vi "Unpack for gRPC.vi"(8 "error in":errorcluster, 9 "configuration / results":enum16{"Configuration", "Results"}(ring), 10 "any":T1, 11 "measurement customizations in":refnum<class "Measurement Plugin.lvclass">) -> (0 "error out":errorcluster, 2 "data value":variant, 3 "measurement customizations out":refnum<class "Measurement Plugin.lvclass">)   [LabVIEW 2021, in "Short-Circuit.lvlib" / "Measurement Plugin.lvclass"]
uses:
  Measurement Plugin.lvclass
  <vilib>/gRPC/LabVIEW gRPC Library/Shared/Any.ctl
  C:/Program Files/National Instruments/LabVIEW 2021/vi.lib/Plug-In SDKs/Measurements/Measurement Plugin Service/Measurement Plugin Service.lvclass
  Measurement Configuration.ctl
  Measurement Results.ctl
  a521b266-ce99-437c-923d-067dcf1e07fd.vi
  3ecd018e-d556-4cbc-bc60-c4ba57204520.vi
  <vilib>/gRPC/LabVIEW gRPC Library/Server API/Translate Protobuf Error.vi
  <vilib>/AdvancedString/1D String Array to Delimited String.vi
  <vilib>/gRPC/LabVIEW gRPC Library/Server API/Server/Get Server DLL Path.vi
  Measurement Plugin.lvclass/Measurement Plugin.ctl
  Short-Circuit.lvlib
  <vilib>/Plug-In SDKs/Measurements/Measurement Plugin Service/Measurement Plugin Service.lvclass
  <vilib>/gRPC/LabVIEW gRPC Library/grpc-lvsupport-release.lvlib
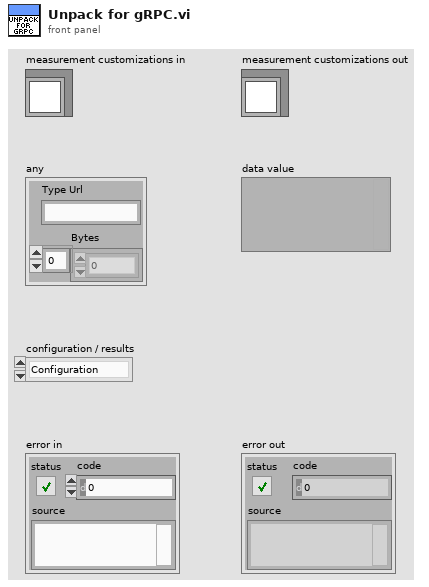
[diagram p1: front panel]
types:
  T1 = typedef "grpc-lvsupport-release.lvlib/Any.ctl" = cluster{"Type Url":string, "Bytes":u8[]}
  T2 = typedef "grpc-lvsupport-release.lvlib/grpcId.ctl" = u64
  T3 = typedef "Short-Circuit.lvlib/Measurement Configuration.ctl" = cluster{"DUT setup time":dbl, "Source delay":dbl, "Aperture time":dbl, "Source resource name":string, "Source sense":i32, "Source current limit":dbl, "Source maximum power":dbl, "Source Voltage (Vo)":dbl, "Load resource name":string, "Load sense":i32, "Load voltage limit range":dbl, "Load Voltage Limit":dbl, "Load Current Level (Io)":dbl, "Switch resource name":string, "Switch - Load Relay Name":string, "Switch - DMM Relay Name":string, "Relay Topology":string, "DMM resource name":string, "DMM Current Range(A)":dbl, "SC - Trigger Delay (sec)":dbl, "SC - Hold Delay (sec)":dbl, "Resolution in Digits":dbl}
  T4 = typedef "Short-Circuit.lvlib/Measurement Results.ctl" = cluster{"Status":string, "Source voltages":dbl[], "Load voltages":dbl[], "Source Current":dbl[], "Load Current":dbl[]}
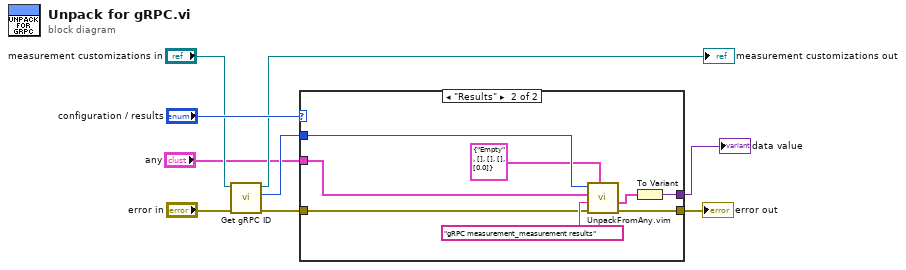
[diagram p0: block diagram]
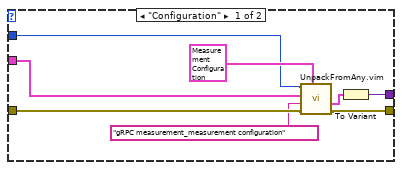
[diagram p2: hidden frame]
diagram:
  n1 = call <vilib>:"Get gRPC ID.vi"("error in"="error in", "measurement plugin service in"="measurement customizations in") -> ("error out"=w6:errorcluster, "gRPC ID"=w3:T2, "measurement plugin service out"=→"measurement customizations out":refnum<class "Measurement Plugin.lvclass">)  [unwired: 7 in]
  n2 = case shown="\"Results\"" "configuration / results" {
    tunnel: w6 -> [w15 w19]
    tunnel: "any" -> [w10 w18]
    tunnel: w3 -> [w12 w22]
    tunnel: [w16 w23] -> w9
    tunnel: [w17 w25] -> w1
    frame "Configuration" {
      n3 = call "UnpackFromAny.vim"("Data Type"=T3 {"DUT setup time"=1.2, "Source delay"=32.0, "Aperture time"=-32.0, "Source resource name"="Lorem ipsum dolor sit", "Source sense"=-64, "Source current limit"=1.0, "Source maximum power"=1.0, "Source Voltage (Vo)"=-32.0, "Load resource name"="", "Load sense"=1009, "Load voltage limit range"=6.0, "Load Voltage Limit"=0.1, "Load Current Level (Io)"=-32.0, "Switch resource name"="", "Switch - Load Relay Name"="", "Switch - DMM Relay Name"="", "Relay Topology"="Configured Topology", "DMM resource name"="", "DMM Current Range(A)"=0.1, "SC - Trigger Delay (sec)"=0.1, "SC - Hold Delay (sec)"=0.1, "Resolution in Digits"=5.5} ("Measurement Configuration"), "error in"=w15, "Message Type"="gRPC measurement_measurement configuration", "Any"=w10, "gRPCid in"=w12) -> ("error out"=w16:errorcluster, "Unpacked Value"=w14:T3)  [unwired: 4 in, 1 out]
      n4 = To Variant(anything=w14) -> (Variant=w17:variant)
    }
    frame "Results" {
      n5 = call "UnpackFromAny.vim"("Data Type"=T4 {"Status"="Empty", "Source voltages"=[], "Load voltages"=[], "Source Current"=[], "Load Current"=[0.0]} ("Measurement Results"), "error in"=w19, "Message Type"="gRPC measurement_measurement results", "Any"=w18, "gRPCid in"=w22) -> ("error out"=w23:errorcluster, "Unpacked Value"=w24:T4)  [unwired: 4 in, 1 out]
      n6 = To Variant(anything=w24) -> (Variant=w25:variant)
    }
  }
  "error out" <- w9
  "data value" <- w1
